vi "DVR.vi"() -> ()   [LabVIEW 2014]
uses:
  <vilib>/Platform/TimedLoop/XDataNode/timing_clust.ctl
  <vilib>/Platform/TimedLoop/XDataNode/nitl_modes.ctl
  <vilib>/Platform/TimedLoop/XDataNode/wakeup.ctl
  <vilib>/platform/TimedLoop/XDataNode/XDataNode.xnode
  <vilib>/Platform/TimedLoop/XDataNode/XDNodeRunTimeDep.lvlib
panel:
  in  "base size":i32=100000
  in  "count":i32=100
  out "dt":dbl=0.17810993525199592
  out "element":dbl=0.6376039460936899
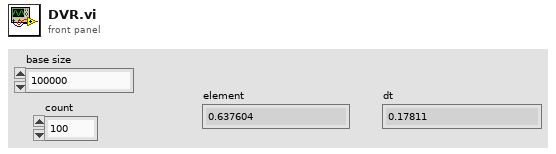
[diagram p1: front panel]
types:
  T1 = typedef "XDNodeRunTimeDep.lvlib/timing_clust.ctl" = cluster{"Expected End [f-1]":u64, "Actual End [f-1]":u64, "Finished Late? [f-1]":bool, "Expected End [i-1]":u64, "Actual End [i-1]":u64, "Finished Late? [i-1]":bool, "Expected Start [i]":u64, "Actual Start [i]":u64, "Expected Start [f]":u64, "Actual Start [f]":u64, "Source Name":string, "Structure Name":string, "Period":i64, "Deadline":i64, "Offset":i64, "Start":i64, "Priority":i32, "Timeout":i32, "Mode":T2, "Wakeup Reason":T3, "Error":errorcluster, "Source Type":string, "Secondary Source Type":string, "Global End Time":u64, "Global Start Time":u64, "Frame Duration":u64, "Iteration Duration":u64, "Assigned CPU":i32, "I/O Scan Engine Mode":u32}
  T2 = typedef "XDNodeRunTimeDep.lvlib/nitl_modes.ctl" = enum32{"No Change", "Process missed periods, maintain original phase", "Discard missed periods, maintain original phase", "Process missed periods, ignore original phase", "Discard missed periods, ignore original phase"}
  T3 = typedef "XDNodeRunTimeDep.lvlib/wakeup.ctl" = enum32{"Normal", "Aborted", "Asynchronous wakeup", "Timing source error", "Timed loop error", "Timeout"}
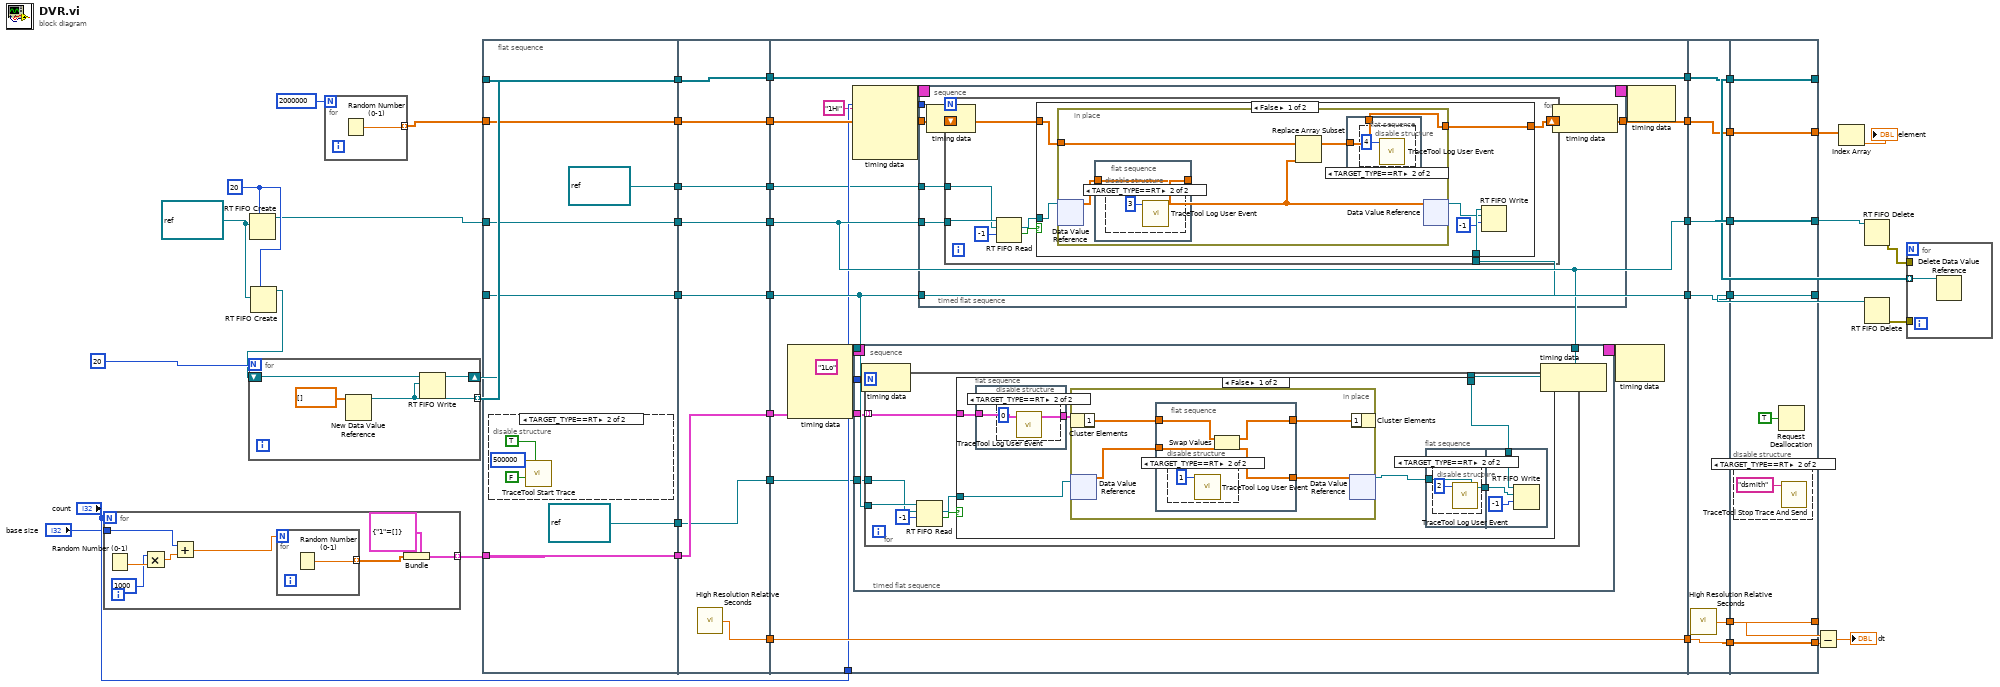
[diagram p0: block diagram]
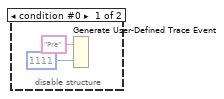
[diagram p2: hidden frame]
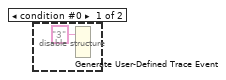
[diagram p3: hidden frame]
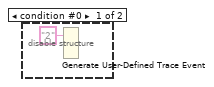
[diagram p4: hidden frame]
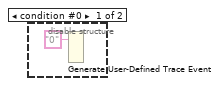
[diagram p6: hidden frame]
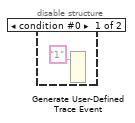
[diagram p7: hidden frame]
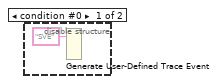
[diagram p8: hidden frame]
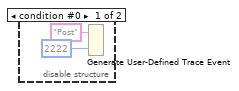
[diagram p10: hidden frame]
diagram:
  w47 = u32 20 ("size (10)")
  w48 = refnum<data-value> refnum ("data value reference")
  n1 = for {
    N: "count" -> [_]
    tunnel: [w55] -> w45 mode=indexing
    tunnel: "base size" -> [w49]
    n2 = Random Number (0-1)() -> (number: 0 to 1=w54:dbl)
    n3 = Multiply(x=1000, y=w54) -> (x*y=w53:dbl)
    n4 = Add(x=w49, y=w53) -> (x+y=w51:dbl)
    n5 = for {
      N: w51 -> [_]
      tunnel: [w57] -> w56 mode=indexing
      n6 = Random Number (0-1)() -> (number: 0 to 1=w57:dbl)
    }
    n7 = Bundle(cluster=cluster{"1":dbl[]} {"1"=[]}, "1"=w56) -> (w55:cluster{"1":dbl[]})
  }
  n8 = RT FIFO Create(1:w48, 4:w47) -> (8:w44:refnum<k33>)  [unwired: 6 in, 2 out]
  n9 = RT FIFO Create(1:w48, 4:w47) -> (8:w27:refnum<k33>)  [unwired: 6 in, 2 out]
  n10 = for {
    N: 20 -> [_]
    tunnel: [w58] -> w37 mode=indexing
    shift-right: [w59] -> w26
    shift-left: w27 -> [w60]
    n11 = New Data Value Reference(data value=dbl[] []) -> (data value reference=w58:refnum<data-value>)  [unwired: 1 in, 1 out]
    n12 = RT FIFO Write(0:w60, 1:w58) -> (8:w59:refnum<k33>)  [unwired: 3 in, 3 out]
  }
  n13 = for {
    N: 2000000 -> [_]
    tunnel: [w62] -> w23 mode=indexing
    n14 = Random Number (0-1)() -> (number: 0 to 1=w62:dbl)
  }
  n15 = flat-sequence {
    tunnel: w23 -> [w65]
    tunnel: w37 -> [w66]
    tunnel: w44 -> [w67]
    tunnel: w26 -> [w68]
    tunnel: w45 -> [w69]
    tunnel: [w69] -> w10
    tunnel: [w68] -> w9
    tunnel: [w67] -> w8
    tunnel: [w66] -> w7
    tunnel: [w65] -> w6
    tunnel: [refnum<data-value> refnum ("element")] -> w4
    tunnel: [refnum<data-value> refnum ("element")] -> w2
    tunnel: [w82] -> w42
    tunnel: [w81] -> w40
    tunnel: [w80] -> w36
    tunnel: [w79] -> w30
    tunnel: [w78] -> w24
    tunnel: [w77] -> w18
    tunnel: w10 -> [w77]
    tunnel: w9 -> [w81]
    tunnel: w8 -> [w82]
    tunnel: w7 -> [w80]
    tunnel: w6 -> [w78]
    tunnel: [w76] -> w5
    tunnel: w4 -> [w76]
    tunnel: [w75] -> w3
    tunnel: w2 -> [w75]
    tunnel: [w93] -> w43
    tunnel: w42 -> [w93]
    tunnel: [w94] -> w41
    tunnel: w40 -> [w94]
    tunnel: w36 -> [w98]
    tunnel: [w98] -> w35
    tunnel: w30 -> [w97]
    tunnel: [w97] -> w29
    tunnel: w24 -> [w96]
    tunnel: [w95] -> w22
    tunnel: "count" -> [w92]
    tunnel: w18 -> [w91]
    tunnel: w5 -> [w84]
    tunnel: w3 -> [w83]
    tunnel: w43 -> [w196]
    tunnel: w41 -> [w195]
    tunnel: w35 -> [w194]
    tunnel: w29 -> [w192]
    tunnel: w22 -> [w191]
    tunnel: [w196] -> w16
    tunnel: [w195] -> w15
    tunnel: [w194] -> w14
    tunnel: [w193] -> w13
    tunnel: [w192] -> w12
    tunnel: [w191] -> w11
    tunnel: [w198] -> w21
    tunnel: [w199] -> w28
    tunnel: [w200] -> w31
    tunnel: [w201] -> w34
    tunnel: [w202] -> w38
    tunnel: [w203] -> w39
    tunnel: w16 -> [w203]
    tunnel: w15 -> [w202]
    tunnel: w14 -> [w201]
    tunnel: w13 -> [w200]
    tunnel: w12 -> [w199]
    tunnel: w11 -> [w198]
    frame #0 {
      n16 = disable-structure shown="TARGET_TYPE==RT" {
        frame condition #0 {
          n17 = Generate User-Defined Trace Event(1:1111 ("trace integer"), 2:"Pre" ("trace string")) -> ()
        }
        frame condition #1 (active) {
          n18 = call <vilib>:"TraceTool Start Trace.vi"("Detailed Tracing? (F)"=TRUE, "VI Tracing? (T)"=FALSE, "Buffer Size (250000 bytes)"=500000) -> ()  [unwired: 7 in, 2 out]
        }
      }
    }
    frame #1 {
      n19 = call <vilib>:"High Resolution Relative Seconds.vi"() -> ("relative seconds"=w79:dbl)
    }
    frame #2 {
      n20 = node-c288("1Lo" ("Structure Name")) -> (w90:T1)  [unwired: 3 in]
      n21 = node-c288("1Hi" ("Structure Name")) -> (w87:T1)  [unwired: 3 in]
      n22 = timed-sequence {
        timing: w90 -> [_]
        timing-out: [_] -> w89
        tunnel: w94 -> [w147]
        tunnel: w93 -> [w146]
        tunnel: w92 -> [w145]
        tunnel: w91 -> [w144]
        tunnel: w83 -> [w143]
        n23 = timed-flat-sequence {
          tunnel: w147 -> [w152]
          tunnel: w146 -> [w151]
          tunnel: w145 -> [w150]
          tunnel: w144 -> [w149]
          tunnel: w143 -> [w148]
          n24 = node-c288() -> ()  [unwired: 1 in, 1 out]
          n25 = for {
            N: w150 -> [_]
            tunnel: w152 -> [w159]
            tunnel: w151 -> [w155]
            tunnel: w149 -> [w154] mode=indexing
            tunnel: w148 -> [w153]
            n26 = RT FIFO Read(0:w159, 1:w153, 2:-1 ("timeout in ms (0)")) -> (9:w156:refnum<data-value>, 10:w157:bool)  [unwired: 1 in, 3 out]
            n27 = case shown="False" w157 {
              tunnel: w156 -> [w165 _]
              tunnel: w155 -> [w164 _]
              tunnel: w154 -> [w162 _]
              frame False {
                n28 = flat-sequence {
                  tunnel: [w166] -> w163
                  tunnel: w162 -> [w166]
                  frame #0 {
                    n29 = disable-structure shown="TARGET_TYPE==RT" {
                      frame condition #0 {
                        n30 = Generate User-Defined Trace Event(2:"0" ("trace string")) -> ()  [unwired: 1 in]
                      }
                      frame condition #1 (active) {
                        n31 = call <vilib>:"TraceTool Log User Event.vi"("Event ID (0-255)"=u32 0) -> ()  [unwired: 10 in, 1 out]
                      }
                    }
                  }
                }
                n32 = in-place {
                  n33 = in-place-cluster #1(w163) -> ("1"=w178:dbl[])
                  n34 = in-place-dvr #2(w165) -> (w177:dbl[])  [unwired: 1 out]
                  n35 = flat-sequence {
                    tunnel: w178 -> [w182]
                    tunnel: w177 -> [w181]
                    tunnel: [w180] -> w176
                    tunnel: [w179] -> w175
                    frame #0 {
                      n36 = disable-structure shown="TARGET_TYPE==RT" {
                        frame condition #0 {
                          n37 = Generate User-Defined Trace Event(2:"SVE" ("trace string")) -> ()  [unwired: 1 in]
                        }
                        frame condition #1 (active) {
                          n38 = call <vilib>:"TraceTool Log User Event.vi"("Event ID (0-255)"=u32 1) -> ()  [unwired: 10 in, 1 out]
                        }
                      }
                      n39 = Swap Values(12:w182, 14:w181) -> (1:w179:dbl[], 3:w180:dbl[])  [unwired: 1 in]
                    }
                  }
                  n40 = in-place-dvr #2(w176) -> (w161:refnum<data-value>)  [unwired: 1 out]
                  n41 = in-place-cluster #1("1"=w175) -> ()  [unwired: 1 out]
                }
                n42 = flat-sequence {
                  tunnel: w161 -> [w169]
                  tunnel: [w169] -> w160
                  tunnel: w164 -> [w173]
                  tunnel: w160 -> [w172]
                  frame #0 {
                    n43 = disable-structure shown="TARGET_TYPE==RT" {
                      frame condition #0 {
                        n44 = Generate User-Defined Trace Event(2:"1" ("trace string")) -> ()  [unwired: 1 in]
                      }
                      frame condition #1 (active) {
                        n45 = call <vilib>:"TraceTool Log User Event.vi"("Event ID (0-255)"=u32 2) -> ()  [unwired: 10 in, 1 out]
                      }
                    }
                  }
                  frame #1 {
                    n46 = RT FIFO Write(0:w173, 1:w172, 2:-1 ("timeout in ms (0)")) -> ()  [unwired: 2 in, 4 out]
                  }
                }
              }
              frame True {
              }
            }
          }
          n47 = node-c288() -> ()  [unwired: 1 in, 1 out]
        }
      }
      n48 = timed-sequence {
        timing: w87 -> [_]
        timing-out: [_] -> w86
        tunnel: w96 -> [w104]
        tunnel: [w103] -> w95
        tunnel: w94 -> [w102]
        tunnel: w93 -> [w101]
        tunnel: w92 -> [w100]
        tunnel: w84 -> [w99]
        n49 = timed-flat-sequence {
          tunnel: w104 -> [w110]
          tunnel: [w109] -> w103
          tunnel: w102 -> [w108]
          tunnel: w101 -> [w107]
          tunnel: w100 -> [w106]
          tunnel: w99 -> [w105]
          n50 = node-c288() -> ()  [unwired: 1 in, 1 out]
          n51 = for {
            N: w106 -> [_]
            shift-right: [w115] -> w109
            shift-left: w110 -> [w114]
            tunnel: w107 -> [w118]
            tunnel: w108 -> [w112]
            tunnel: w105 -> [w111]
            n52 = RT FIFO Read(0:w118, 1:w111, 2:-1 ("timeout in ms (0)")) -> (9:w113:refnum<data-value>, 10:w116:bool)  [unwired: 1 in, 3 out]
            n53 = case shown="False" w116 {
              tunnel: [w122 w136] -> w115
              tunnel: w114 -> [w123 w136]
              tunnel: w113 -> [w124 _]
              tunnel: w112 -> [w121 _]
              frame False {
                n54 = in-place {
                  in-place-border: w123 -> [w126]
                  in-place-border: [w128] -> w122
                  n55 = in-place-dvr #3(w124) -> (w129:dbl[])  [unwired: 1 out]
                  n56 = flat-sequence {
                    tunnel: w129 -> [w133]
                    tunnel: [w133] -> w125
                    frame #0 {
                      n57 = disable-structure shown="TARGET_TYPE==RT" {
                        frame condition #0 {
                          n58 = Generate User-Defined Trace Event(2:"2" ("trace string")) -> ()  [unwired: 1 in]
                        }
                        frame condition #1 (active) {
                          n59 = call <vilib>:"TraceTool Log User Event.vi"("Event ID (0-255)"=u32 3) -> ()  [unwired: 10 in, 1 out]
                        }
                      }
                    }
                  }
                  n60 = Replace Array Subset(array=w126, new element=w125) -> (w127:dbl[])  [unwired: 1 in]
                  n61 = flat-sequence {
                    tunnel: [w130] -> w128
                    tunnel: w127 -> [w130]
                    frame #0 {
                      n62 = disable-structure shown="TARGET_TYPE==RT" {
                        frame condition #0 {
                          n63 = Generate User-Defined Trace Event(2:"3" ("trace string")) -> ()  [unwired: 1 in]
                        }
                        frame condition #1 (active) {
                          n64 = call <vilib>:"TraceTool Log User Event.vi"("Event ID (0-255)"=u32 4) -> ()  [unwired: 10 in, 1 out]
                        }
                      }
                    }
                  }
                  n65 = in-place-dvr #3(w125) -> (w120:refnum<data-value>)  [unwired: 1 out]
                }
                n66 = RT FIFO Write(0:w121, 1:w120, 2:-1 ("timeout in ms (0)")) -> ()  [unwired: 2 in, 4 out]
              }
              frame True {
              }
            }
          }
          n67 = node-c288() -> ()  [unwired: 1 in, 1 out]
        }
      }
      n68 = node-c288(w89) -> ()  [unwired: 1 out]
      n69 = node-c288(w86) -> ()  [unwired: 1 out]
    }
    frame #3 {
      n70 = call <vilib>:"High Resolution Relative Seconds.vi"() -> ("relative seconds"=w193:dbl)
    }
    frame #4 {
      n71 = disable-structure shown="TARGET_TYPE==RT" {
        frame condition #0 {
          n72 = Generate User-Defined Trace Event(1:2222 ("trace integer"), 2:"Post" ("trace string")) -> ()
        }
        frame condition #1 (active) {
          n73 = call <vilib>:"TraceTool Stop Trace And Send.vi"("Trace Host Network Address"="dsmith") -> ()  [unwired: 10 in, 1 out]
        }
      }
      n74 = Request Deallocation(TRUE ("flag")) -> ()
    }
  }
  n75 = Subtract(x=w31, y=w28) -> (x-y=→"dt":dbl)
  n76 = Index Array(array=w21) -> (element=→"element":dbl)  [unwired: 1 in]
  n77 = RT FIFO Delete(0:w39) -> (11:w32:errorcluster)  [unwired: 2 in]
  n78 = RT FIFO Delete(0:w38) -> (11:w33:errorcluster)  [unwired: 2 in]
  n79 = for {
    tunnel: w34 -> [w207] mode=indexing
    tunnel: w33 -> [_]
    tunnel: w32 -> [_]
    n80 = Delete Data Value Reference(data value reference=w207) -> ()  [unwired: 1 in, 2 out]
  }
